vi "Get Position (SubVI).vi"(6 "Device Address In":i32, 7 "Motor":i32, 8 "entrée d'erreur (pas d'erreur)":errorcluster, 9 "DeviceKey In":string, 10 "pos":i32, 11 "Refnum de .NET en entrée":refnum<k24>) -> (0 "sortie d'erreur":errorcluster, 1 "Device Address Out":i32, 2 "Position":i32, 3 "Refnum de .NET en sortie":refnum<k24>, 5 "DeviceKey Out":string)   [LabVIEW 2017]
doc: "by Tanguy BOULARD"
uses:
  dll/CmdLib.dll
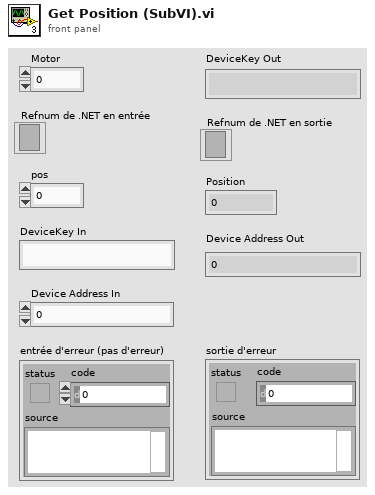
[diagram p1: front panel]
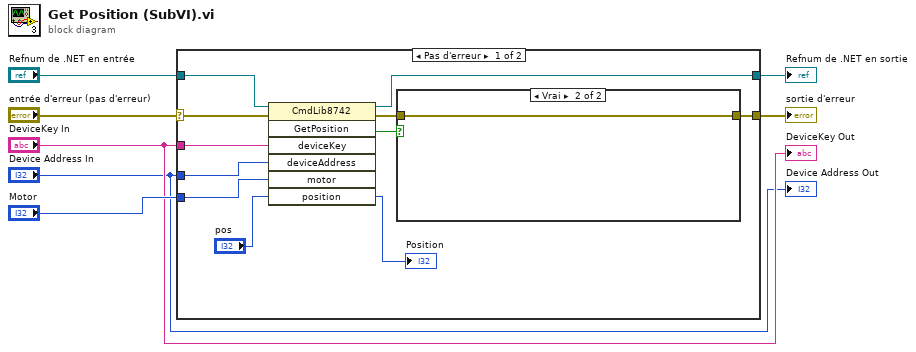
[diagram p0: block diagram]
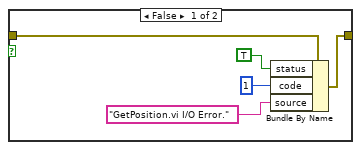
[diagram p2: hidden frame]
diagram:
  n1 = case shown="Pas d'erreur" "entrée d'erreur (pas d'erreur)" {
    selector: "entrée d'erreur (pas d'erreur)" -> [w15 w25]
    tunnel: "Refnum de .NET en entrée" -> [w18 w26]
    tunnel: [w17 w26] -> w4
    tunnel: "Motor" -> [w11 _]
    tunnel: "DeviceKey In" -> [w16 _]
    tunnel: [w12 w25] -> w6
    tunnel: "Device Address In" -> [w10 _]
    frame No Error {
      n2 = invoke class="CmdLib8742" method="GetPosition"(reference=w18, error in=w15, "deviceKey"=w16, "deviceAddress"=w10, "motor"=w11, "position"="pos") -> (reference out=w17:refnum<k24>, error out=w13:errorcluster, "GetPosition"=w14:bool, "position"=→"Position":i32)  [unwired: 1 in, 3 out]
      n3 = case shown="Vrai" w14 {
        tunnel: w13 -> [w23 w24]
        tunnel: [w22 w24] -> w12
        frame False {
          n4 = Bundle By Name(cluster=w23, "status"=TRUE, "code"=1, "source"="GetPosition.vi I/O Error.") -> (w22:errorcluster)
        }
        frame True {
        }
      }
    }
    frame Error {
    }
  }
  "sortie d'erreur" <- w6
  "Refnum de .NET en sortie" <- w4
  "DeviceKey Out" <- "DeviceKey In"
  "Device Address Out" <- "Device Address In"
